vi "Video File Frame Read.vi"(8 "error in (no error)":errorcluster, 10 "Image Dst":T1, 11 "Video File in":refnum<class "Video File.lvclass">) -> (0 "error out":errorcluster, 2 "Video Frame out":refnum<class "Video Frame.lvclass">, 3 "Video File out":refnum<class "Video File.lvclass">, 4 "Playback Finished?":bool, 6 "Looped?":bool)   [LabVIEW 2018, in "Video File.lvclass"]
uses:
  Video File.lvclass
  <vilib>/vision/Image Controls.llb/IMAQ Image.ctl
  Video Frame/Video Frame.lvclass
  Video File.lvclass/Video File.ctl
  ROIed Video Frame/ROIed Video Frame.lvclass
  C:/Users/aaron.jencks/Documents/GitHub/emerson_seed_object_detection/LabVIEW/Projects/Paul's Video Viewer/Classes/Video Frame/Video Frame.lvclass
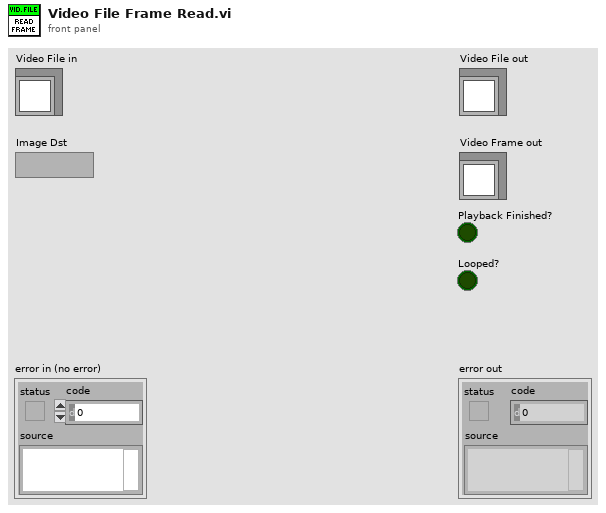
[diagram p1: front panel]
types:
  T1 = typedef "IMAQ Image.ctl" = refnum<image>
  T2 = typedef "IMAQ AVI2 Refnum.ctl" = refnum<k20>
  T3 = cluster{"Width":u32, "Height":u32, "Frames Per Second":u32, "Codec":string, "Has Data":bool}
  T4 = cluster{"Global Rectangle":i32[], "Contours":cluster{"Contour Type":u32, "ROI Type":u32, "Points":i32[]}[]}
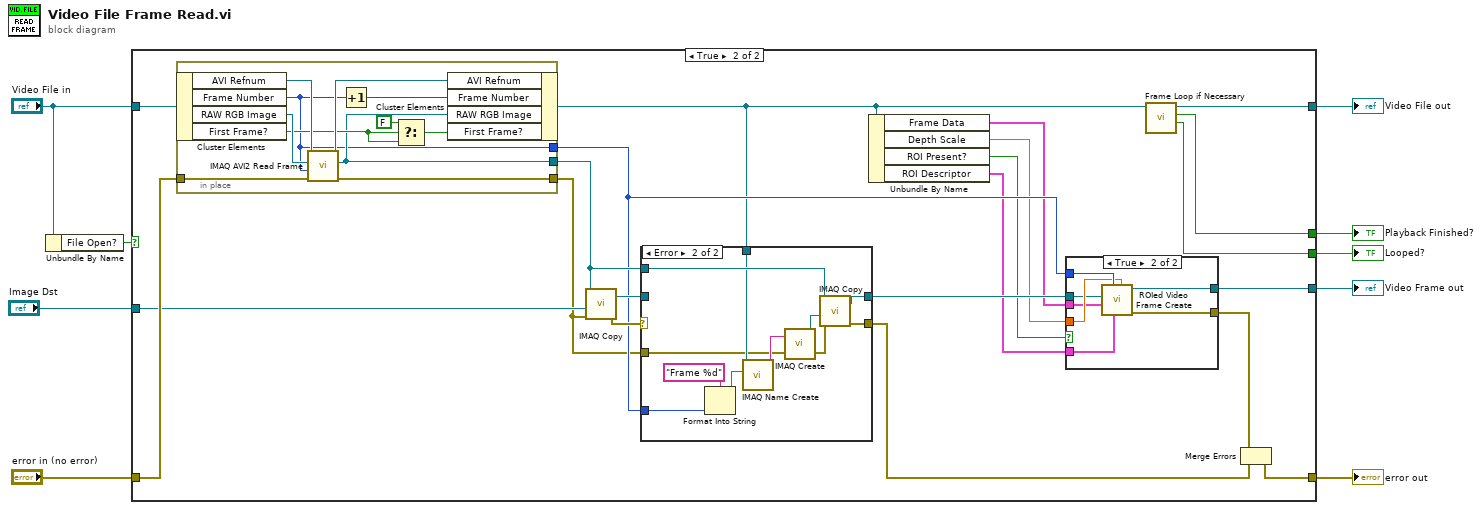
[diagram p0: block diagram]
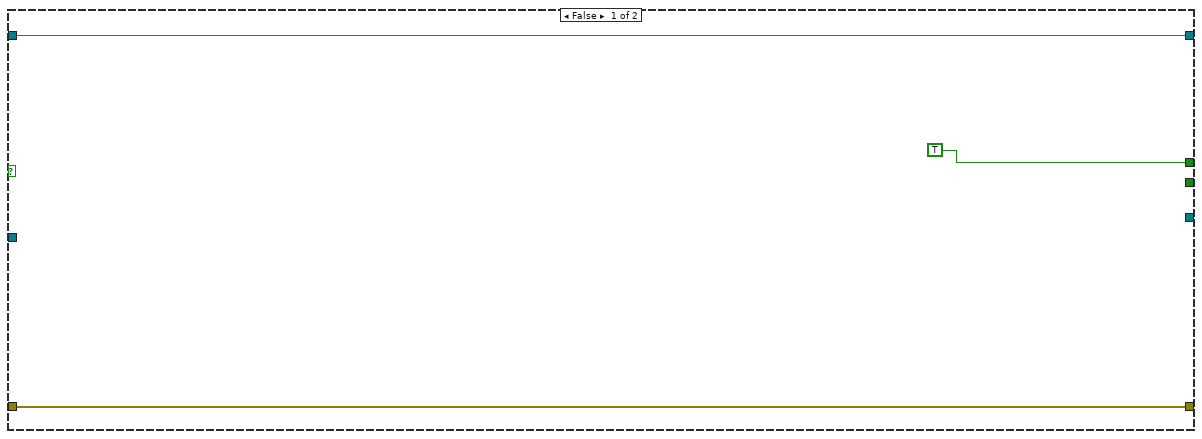
[diagram p2: hidden frame]
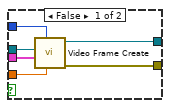
[diagram p3: hidden frame]
diagram:
  n1 = Unbundle By Name("Video File in") -> ("File Open?"=w4:bool)
  n2 = case shown="True" w4 {
    tunnel: "error in (no error)" -> [w11 w33]
    tunnel: [w11 w13] -> w8
    tunnel: [w12 w21] -> w7
    tunnel: "Image Dst" -> [_ w32]
    tunnel: "Video File in" -> [w12 w28]
    tunnel: [_ w23] -> w3
    tunnel: [TRUE ("Finished?") w20] -> w2
    tunnel: [_ w19] -> w1
    frame False {
    }
    frame True {
      n3 = in-place {
        in-place-border: w33 -> [w67]
        in-place-border: [w62] -> w16
        in-place-border: [w61] -> w29
        in-place-border: [w60] -> w26
        n4 = in-place-cluster #1(w28) -> ("AVI Refnum"=w70:T2, "Frame Number"=w60:u32, "RAW RGB Image"=w68:T1, "First Frame?"=w65:bool)
        n5 = call "IMAQ AVI2 Read Frame"("error in (no error)"=w67, "Frame Number"=w60, "Image"=w68, "AVI Refnum"=w70) -> ("error out"=w62:errorcluster, "Image Out"=w61:T1, "AVI Refnum (duplicate)"=w69:T2)  [unwired: 5 out]
        n6 = Increment(x=w60) -> (x+1=w66:u32)
        n7 = Select(t=FALSE, s=w65, f=w65) -> (s? t:f=w63:bool)
        n8 = in-place-cluster #1("AVI Refnum"=w69, "Frame Number"=w66, "RAW RGB Image"=w61, "First Frame?"=w63) -> (w22:refnum<class "Video File.lvclass">)
      }
      n9 = call "IMAQ Copy"("error in (no error)"=w16, "Image Dst"=w32, "Image Src"=w29) -> ("error out"=w31:errorcluster, "Image Dst Out"=w30:T1)  [unwired: 3 in]
      n10 = case shown="Error" w31 {
        selector: w31 -> [w47 _]
        tunnel: w30 -> [w48 _]
        tunnel: [w48 w55] -> w27
        tunnel: w29 -> [_ w59]
        tunnel: [w47 w56] -> w14
        tunnel: w22 -> [_ w54]
        tunnel: w26 -> [_ w50]
        tunnel: w16 -> [_ w49]
        frame No Error {
        }
        frame Error {
          n11 = Format Into String(format string="Frame %d", w50) -> (resulting string=w52:string)  [unwired: 2 in, 1 out]
          n12 = call "IMAQ Name Create.vi"("Name (\"\")"=w52, "Video File in"=w54) -> ("Name Out"=w53:string)  [unwired: 7 in, 2 out]
          n13 = call "IMAQ Create"("Image Name"=w53, "error in (no error)"=w49) -> ("New Image"=w58:T1, "error out"=w57:errorcluster)  [unwired: 3 in]
          n14 = call "IMAQ Copy"("error in (no error)"=w57, "Image Dst"=w58, "Image Src"=w59) -> ("error out"=w56:errorcluster, "Image Dst Out"=w55:T1)  [unwired: 3 in]
        }
      }
      n15 = Unbundle By Name(w22) -> ("Frame Data"=w25:T3, "Depth Scale"=w24:dbl, "ROI Present?"=w18:bool, "ROI Descriptor"=w17:T4)
      n16 = case shown="True" w18 {
        tunnel: w27 -> [w39 w44]
        tunnel: w26 -> [w38 w46]
        tunnel: w25 -> [w37 w43]
        tunnel: w24 -> [w36 w45]
        tunnel: [w35 w41] -> w23
        tunnel: w17 -> [_ w42]
        tunnel: [w34 w40] -> w15
        frame False {
          n17 = call "Video Frame Create.vi"("Depth Scale"=w36, "Frame Number"=w38, "Frame Data"=w37, "Image Dst"=w39) -> ("error out"=w34:errorcluster, "Video Frame out"=w35:refnum<class "Video Frame.lvclass">)  [unwired: 6 in]
        }
        frame True {
          n18 = call "ROIed Video Frame Create.vi"("Depth Scale"=w45, "ROI Descriptor"=w42, "Frame Number"=w46, "Frame Data"=w43, "Image Dst"=w44) -> ("error out"=w40:errorcluster, "ROIed Video Frame out"=w41:refnum<class "ROIed Video Frame.lvclass">)  [unwired: 5 in]
        }
      }
      n19 = call-dynamic "Frame Loop if Necessary.vi"("Video File in"=w22) -> ("Looped?"=w19:bool, "Finished?"=w20:bool, "Video File out"=w21:refnum<class "Video File.lvclass">)  [unwired: 7 in, 1 out]
      n20 = Merge Errors(w15, w14) -> (w13:errorcluster)
    }
  }
  "error out" <- w8
  "Video File out" <- w7
  "Video Frame out" <- w3
  "Playback Finished?" <- w2
  "Looped?" <- w1
